vi "Modify Event.vi"(8 "error in (no error)":errorcluster, 9 "EventIndex":i32, 10 "Event":T1, 11 "Tosca in":refnum<class "Parameters.lvclass">) -> (0 "error out":errorcluster, 3 "Tosca out":refnum<class "Parameters.lvclass">)   [LabVIEW 2020, in "Parameters.lvclass"]
uses:
  Parameters.lvclass
  Digital Input VIs/Tosca-Input Event.ctl
  Digital Input VIs/Tosca-Input Criterion.ctl
  epl-vi-lib/Utility VIs/Type Defs/Logic State.ctl
  Typedefs/Tosca-Accumulator.ctl
  Parameters.lvclass/Parameters.ctl
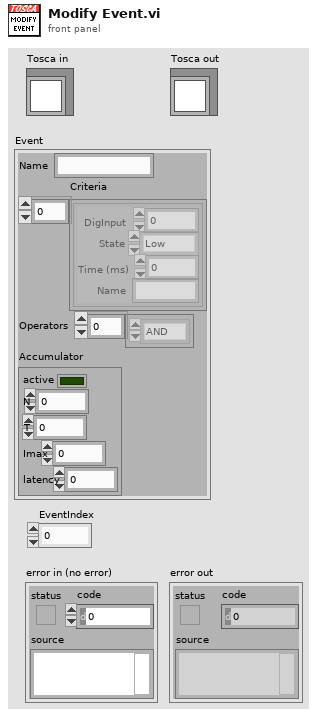
[diagram p1: front panel]
types:
  T1 = typedef "Tosca-Input Event.ctl" = cluster{"Name":string, "Criteria":T2[], "Operators":enum16{"AND", "OR"}[], "Accumulator":T4}
  T2 = typedef "Tosca-Input Criterion.ctl" = cluster{"DigInput":i32, "State":T3, "Time (ms)":i32, "Name":string}
  T3 = typedef "Logic State.ctl" = enum16{"Low", "High", "Rising", "Falling"}
  T4 = typedef "Tosca-Accumulator.ctl" = cluster{"active":bool, "N":i32, "T":dbl, "Imax":dbl, "latency":dbl}
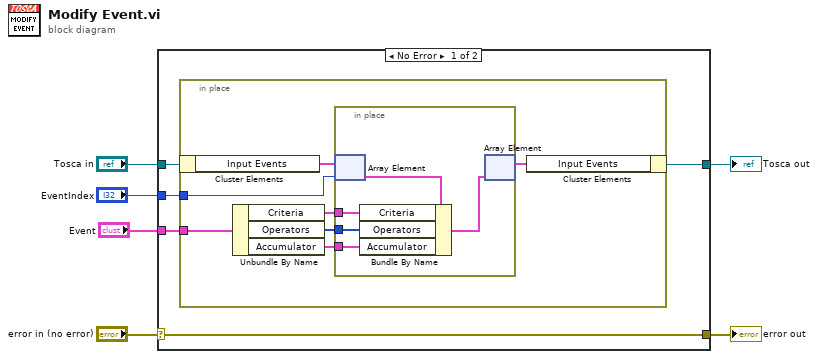
[diagram p0: block diagram]
diagram:
  n1 = case shown="No Error" "error in (no error)" {
    selector: "error in (no error)" -> [w11 w25]
    tunnel: [w11 w25] -> w5
    tunnel: [w9 w24] -> w3
    tunnel: "Tosca in" -> [w10 w24]
    tunnel: "EventIndex" -> [w8 _]
    tunnel: "Event" -> [w7 _]
    frame No Error {
      n2 = in-place {
        in-place-border: w8 -> [w16]
        in-place-border: w7 -> [w15]
        n3 = in-place-cluster #1(w10) -> ("Input Events"=w18:T1[])
        n4 = Unbundle By Name(w15) -> ("Criteria"=w14:T2[], "Operators"=w13:enum16{"AND", "OR"}[], "Accumulator"=w12:T4)
        n5 = in-place {
          in-place-border: w14 -> [w21]
          in-place-border: w13 -> [w20]
          in-place-border: w12 -> [w19]
          n6 = in-place-array #2(w18, w16) -> (w23:T1)
          n7 = Bundle By Name(cluster=w23, "Criteria"=w21, "Operators"=w20, "Accumulator"=w19) -> (w22:T1)
          n8 = in-place-array #2(w22) -> (w17:T1[])  [unwired: 1 out]
        }
        n9 = in-place-cluster #1("Input Events"=w17) -> (w9:refnum<class "Parameters.lvclass">)
      }
    }
    frame Error {
    }
  }
  "error out" <- w5
  "Tosca out" <- w3
